vi "Save Image.vi"(8 "error in (no error)":errorcluster, 11 "Save Image in":refnum<class "Save Image.lvclass">) -> (0 "error out":errorcluster, 3 "Save Image out":refnum<class "Save Image.lvclass">)   [LabVIEW 2018, in "Save Image.lvclass"]
doc: "Save image using the Python Toolkit"
uses:
  Save Image.lvclass
  Save Image.lvclass/Save Image.ctl
  Channel/Channel.lvclass/Channel.ctl
  Log File/CCS_Log File.lvclass/CCS_Log File.ctl
  Keywords Log File/Keywords Log File.lvclass
  C:/Users/Denis/Desktop/S4CCS/S4CCS/Log File/CCS_Log File.lvclass
  State Machine/CCS_State Machine.lvclass
  RxTx/CCS_RxTx.lvclass
  Simulated_CCD_Camera/Simulated Camera.lvclass
  Header content/Header content.lvclass
  Log File/CCS_Log File.lvclass
  Error log/Error log.lvclass
  Channel/Channel.lvclass
  Python Toolkit/Python Toolkit.lvclass
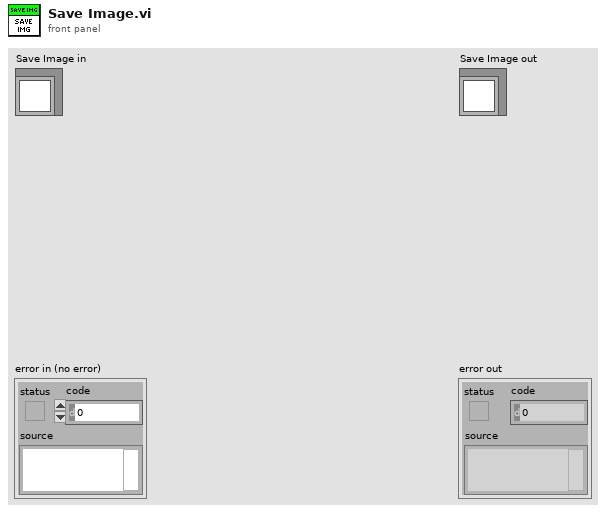
[diagram p1: front panel]
types:
  T1 = cluster{"CCD":string, "S4GUI":string, "S4ICS":string, "TCS":string, "FOCUSER":string, "WSTATION":string, "GENERAL KW":string}
  T2 = cluster{"Image path":path, "Remote IP":string, "Channel":u8, "ACS mode":u16, "Communication":u16}
  T3 = cluster{"State Machine.lvclass":refnum<class "CCS_State Machine.lvclass">, "RxTx.lvclass":refnum<class "CCS_RxTx.lvclass">, "Simulated_CCD_Camera.lvclass":refnum<class "Simulated Camera.lvclass">, "Save_Header_RxTx.lvclass":refnum<class "CCS_RxTx.lvclass">, "Header Content.lvclass":refnum<class "Header content.lvclass">, "Status SM.lvclass":refnum<class "CCS_State Machine.lvclass">, "Status RxTx.lvclass":refnum<class "CCS_RxTx.lvclass">, "Log File.lvclass":refnum<class "CCS_Log File.lvclass">, "Error log.lvclass":refnum<class "Error log.lvclass">, "Keywords Log File.lvclass":refnum<class "Keywords Log File.lvclass">}
  T4 = cluster{"CYCLES_DONE":u16, "LAST_IMAGE_NAME":string, "DISK_SPACE":u16, "FRAMES_DONE":u16, "CCD_STATUS":string, "CURRENT_TEMPERATURE":i16, "TEMPERATURE_STATUS":string, "FRAME_EXPOSURE_TIME":sgl, "ERROR":bool, "SERIAL_NUMBER":u16, "ACQUIRING":bool, "IMAGE_INDEX":u32, "SEQS_DONE":u16}
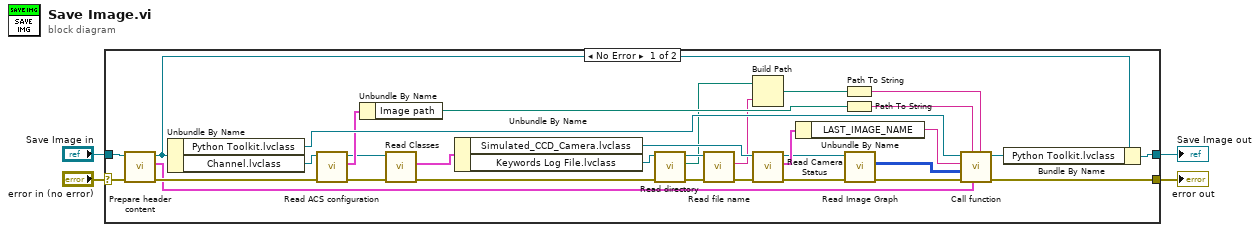
[diagram p0: block diagram]
diagram:
  n1 = case shown="No Error" "error in (no error)" {
    selector: "error in (no error)" -> [w26 w37]
    tunnel: [w33 w37] -> w1
    tunnel: [w36 w38] -> w2
    tunnel: "Save Image in" -> [w28 w38]
    frame No Error {
      n2 = call "Prepare header content.vi"("error in (no error)"=w26, "Save Image in"=w28) -> ("error out"=w24:errorcluster, "cluster of jsons 2"=w18:T1, "Save Image out"=w27:refnum<class "Save Image.lvclass">)  [unwired: 7 in]
      n3 = Unbundle By Name(w27) -> ("Python Toolkit.lvclass"=w35:refnum<class "Python Toolkit.lvclass">, "Channel.lvclass"=w25:refnum<class "Channel.lvclass">)
      n4 = call-dynamic "Read ACS configuration.vi"("error in (no error)"=w24, "Channel in"=w25) -> ("error out"=w16:errorcluster, "acs init configuration"=w23:T2, "Channel out"=w17:refnum<class "Channel.lvclass">)  [unwired: 7 in]
      n5 = Unbundle By Name(w23) -> ("Image path"=w22:path)
      n6 = call "Read Classes.vi"("error in (no error)"=w16, "Channel in"=w17) -> ("error out"=w15:errorcluster, "Classes"=w14:T3)  [unwired: 7 in, 1 out]
      n7 = Unbundle By Name(w14) -> ("Simulated_CCD_Camera.lvclass"=w12:refnum<class "Simulated Camera.lvclass">, "Keywords Log File.lvclass"=w13:refnum<class "Keywords Log File.lvclass">)
      n8 = call "Read directory.vi"("error in (no error)"=w15, "Log File in"=w13) -> ("error out"=w11:errorcluster, "directory"=w8:path, "Log File out"=w9:refnum<class "Keywords Log File.lvclass">)  [unwired: 7 in]
      n9 = call "Read file name.vi"("error in (no error)"=w11, "Log File in"=w9) -> ("error out"=w10:errorcluster, "file name"=w7:string)  [unwired: 7 in, 1 out]
      n10 = Build Path(base path=w8, name or relative path=w7) -> (appended path=w6:path)
      n11 = call "Read Camera Status.vi"("error in (no error)"=w10, "CCDCamera in"=w12) -> ("error out"=w30:errorcluster, "Camera Status"=w31:T4, "CCDCamera out"=w29:refnum<class "Simulated Camera.lvclass">)  [unwired: 7 in]
      n12 = Unbundle By Name(w31) -> ("LAST_IMAGE_NAME"=w20:string)
      n13 = Path To String(path=w6) -> (string=w5:string)
      n14 = Path To String(path=w22) -> (string=w21:string)
      n15 = call "Read Image Graph.vi"("error in (no error)"=w30, "CCDCamera in"=w29) -> ("error out"=w32:errorcluster, "Image Graph"=w19:u16[][])  [unwired: 7 in, 1 out]
      n16 = call "Call function.vi"("log file path"=w5, "cluster of jsons"=w18, "night dir"=w21, "error in (no error)"=w32, "Array"=w19, "file name"=w20, "Python Toolkit in"=w35) -> ("error out"=w33:errorcluster, "Python Toolkit out"=w34:refnum<class "Python Toolkit.lvclass">)  [unwired: 3 in]
      n17 = Bundle By Name(cluster=w27, "Python Toolkit.lvclass"=w34) -> (w36:refnum<class "Save Image.lvclass">)
    }
    frame Error {
    }
  }
  "error out" <- w1
  "Save Image out" <- w2
